vi "StateMachineDAQ-modified.vi"() -> ()   [LabVIEW 2015]
doc: "Use this template to build a user interface event handler design pattern. Use this pattern for dialog boxes and other user interfaces. You also can create and execute user-defined events that the VI can handle the same way as user interface events."
uses:
  StateMachineDAQState.ctl
  <vilib>/Utility/error.llb/DialogType.ctl
  <vilib>/DAQmx/read.llb/DAQmx Read (Analog Wfm 1Chan NSamp).vi
  <vilib>/DAQmx/create/channels.llb/DAQmx Create Channel (AI-Voltage-Basic).vi
  <vilib>/DAQmx/configure/timing.llb/DAQmx Timing (Sample Clock).vi
  <vilib>/DAQmx/miscellaneous.llb/DAQmx Fill In Error Info.vi
  <resource>/objmgr/daqmx.rc
panel:
  in  "Process 1":bool
  in  "File Path":path
  in  "Acquire Data":bool
  in  "Log Data":bool
  in  "File Comment":string
  in  "DAQ Parameters":T1={"physical channels"="", "maximum value"=5.0, "minimum value"=-5.0, "rate"=1000.0, "read period"=0.5} {"read period" format="%0.2f"; "rate" format="%0.2f"; "minimum value" format="%0.2f"; "maximum value" format="%0.2f"}
  out "Waveform Chart":waveform(dbl)(graph)
  in  "quit":bool
  # "V"
  # "V"
  # "Hz"
  # "s"
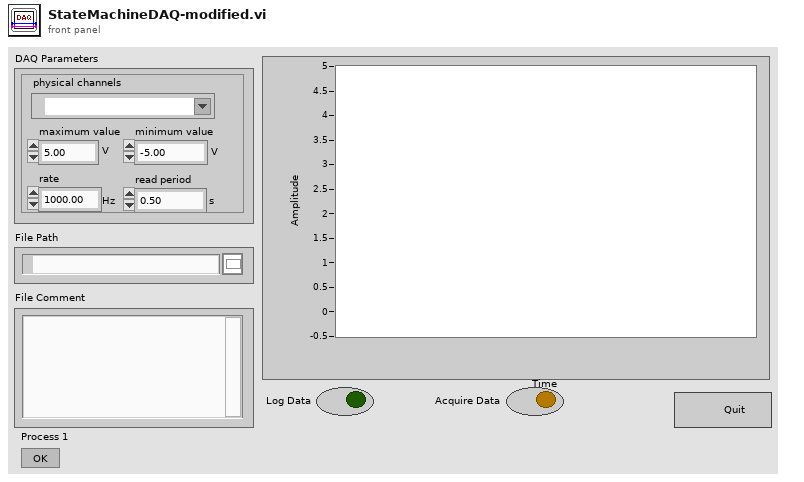
[diagram p1: front panel]
types:
  T1 = cluster{"physical channels":tag, "maximum value":dbl, "minimum value":dbl, "rate":dbl, "read period":dbl}
  T2 = typedef "StateMachineDAQState.ctl" = enum16{"Init", "Idle", "CheckError", "Finalize", "ConfigDAQ", "StartDAQ", "AcquireAndLog", "StopDAQ", "ClearDAQ", "OpenFile", "CloseFile", "Process 1"}
  T3 = typedef "DialogType.ctl" = u16
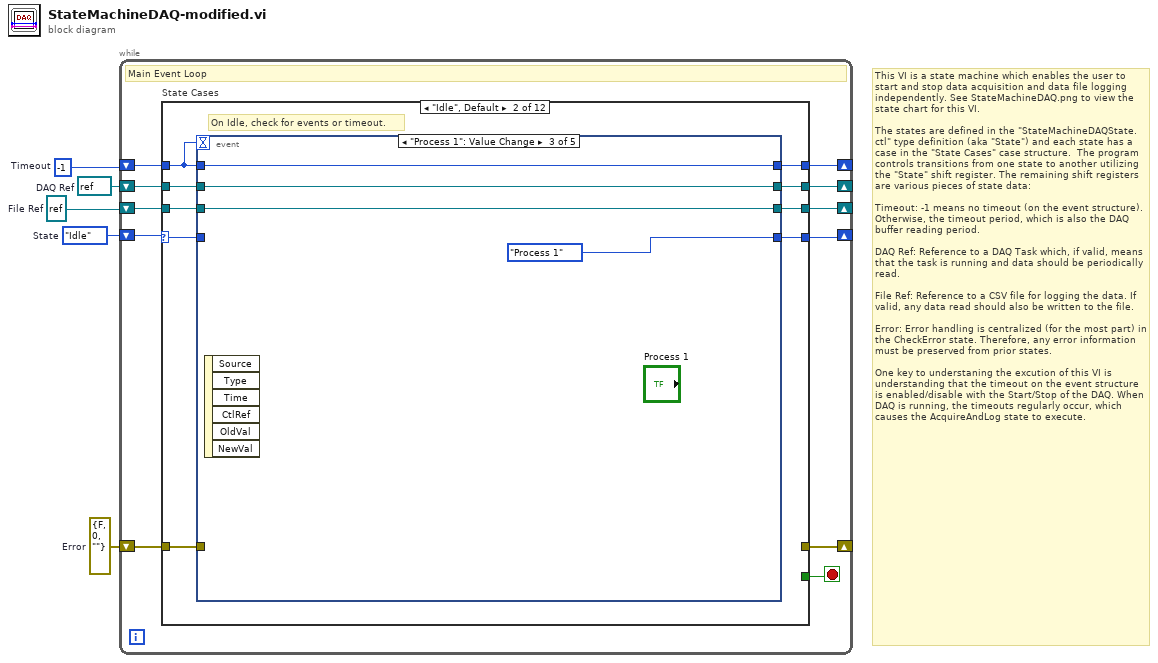
[diagram p0: block diagram]
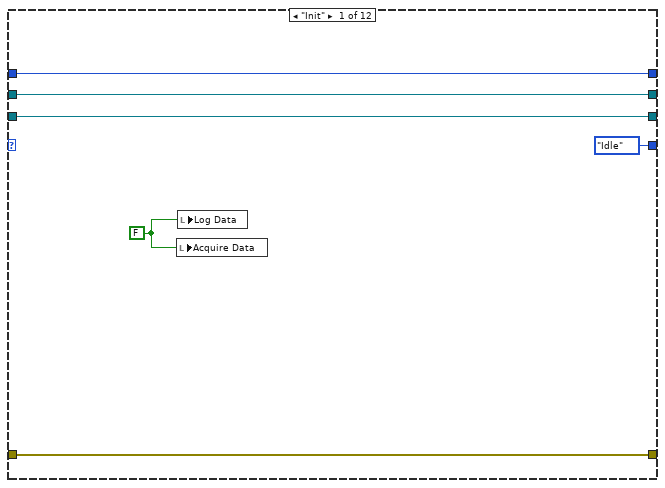
[diagram p2: hidden frame]
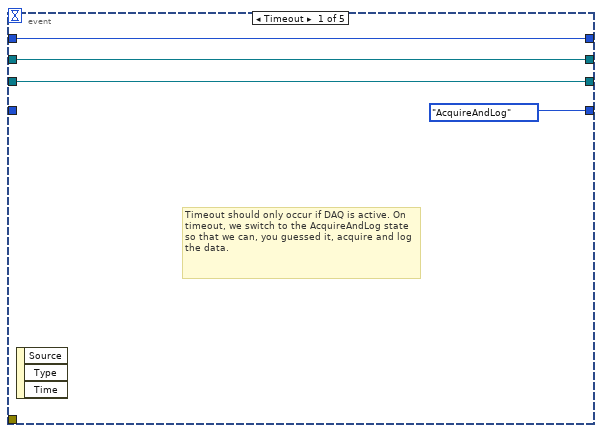
[diagram p3: hidden frame]
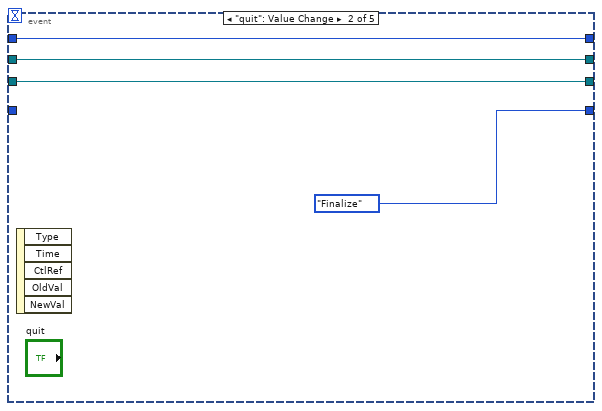
[diagram p4: hidden frame]
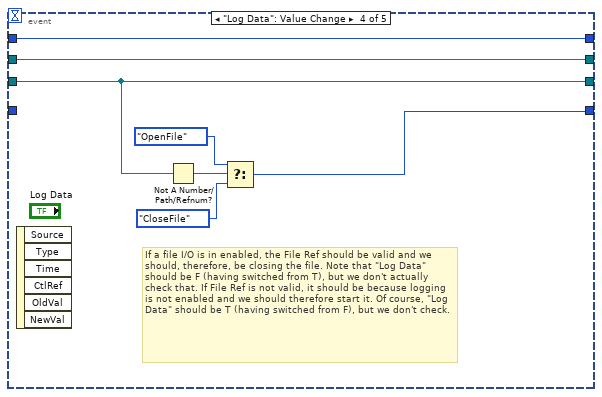
[diagram p5: hidden frame]
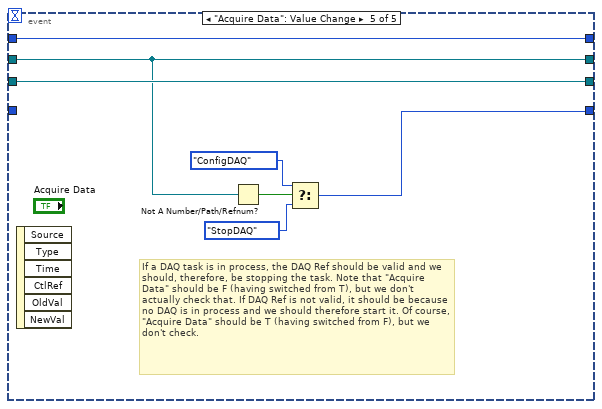
[diagram p6: hidden frame]
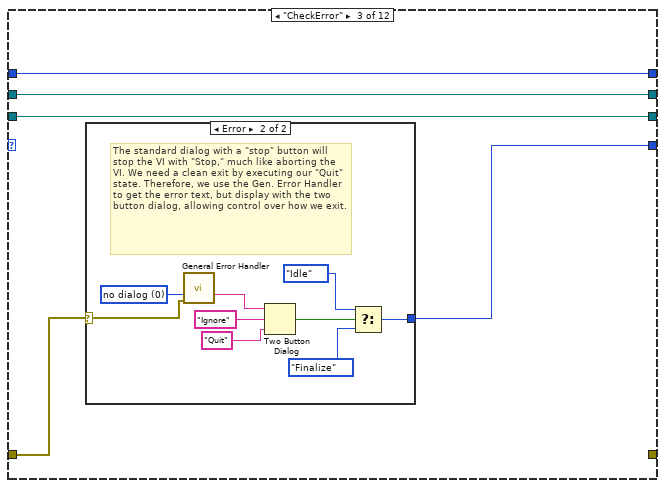
[diagram p7: hidden frame]
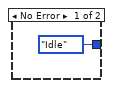
[diagram p8: hidden frame]
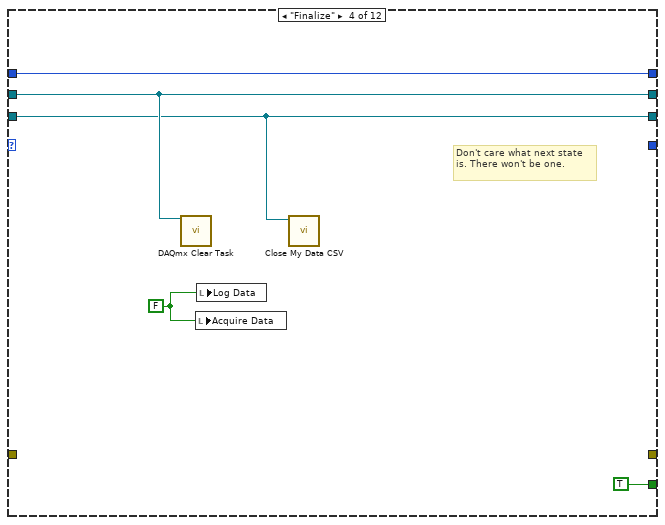
[diagram p9: hidden frame]
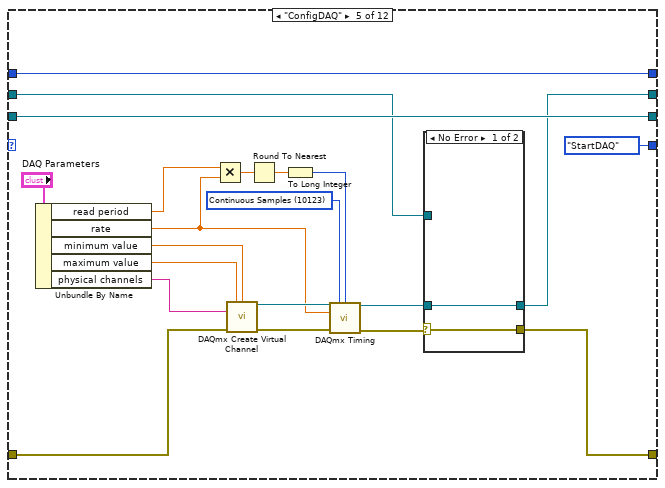
[diagram p10: hidden frame]
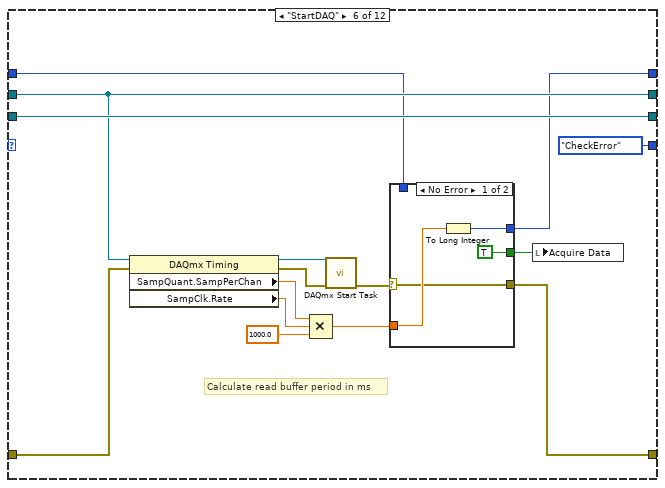
[diagram p12: hidden frame]
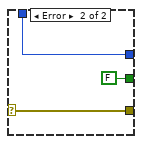
[diagram p13: hidden frame]
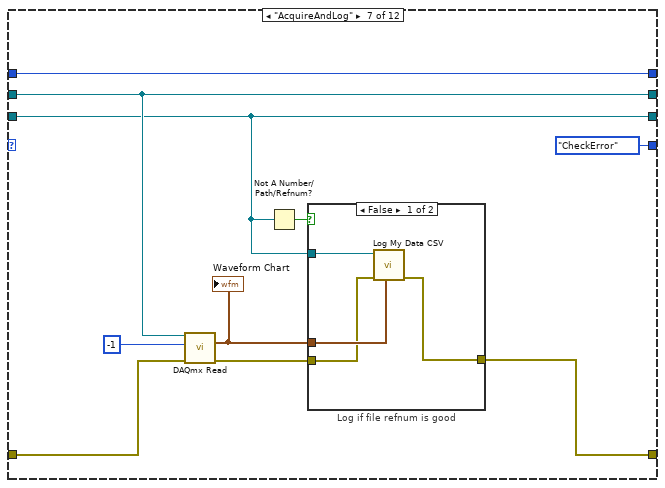
[diagram p14: hidden frame]
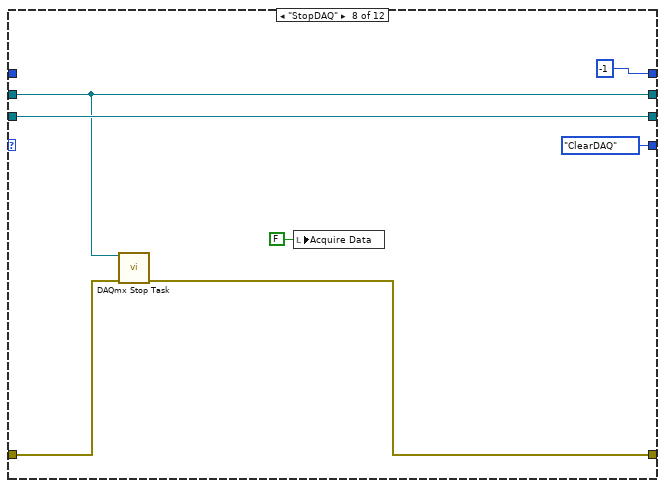
[diagram p16: hidden frame]
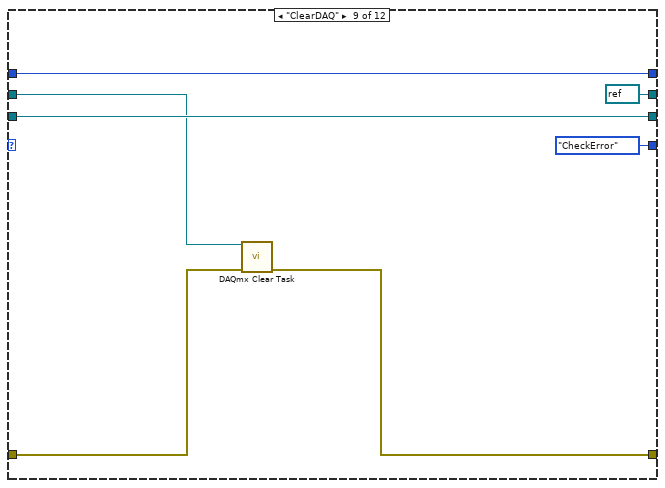
[diagram p17: hidden frame]
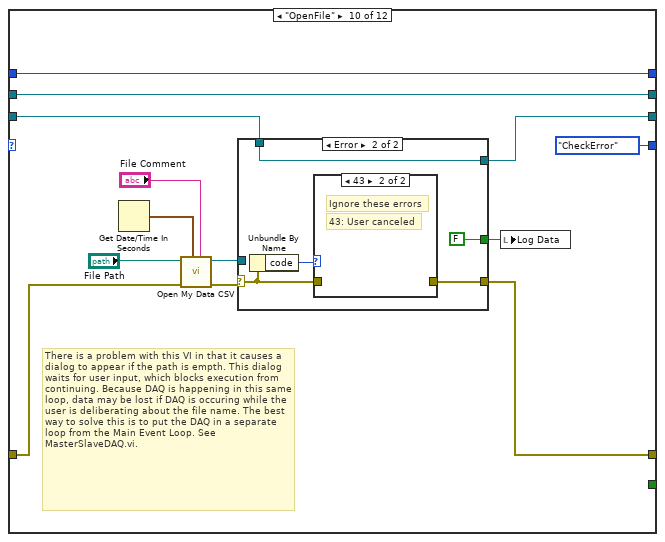
[diagram p18: hidden frame]
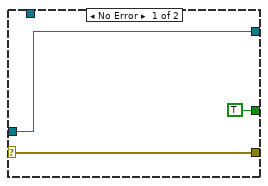
[diagram p19: hidden frame]
diagram:
  w1 = errorcluster {"status"=FALSE, "code"=0, "source"=""}  # Error
  w2 = refnum<file> refnum  # File Ref
  w3 = refnum<k21> refnum  # DAQ Ref
  w4 = StateMachineDAQState."Idle"  # State
  w5 = -1  # Timeout
  # "This VI is a state machine which enables the user to start and stop data acquisition and data file logging independently. See StateMachineDAQ.png to view the state chart for this VI.\n\nThe states are defined in the \"StateMachineDAQState.ctl\" type definition (aka \"State\") and each state has a case in the \"State Cases\" case structure.  The program controls transitions from one state to another utilizing the \"State\" shift register. The remaining shift registers are various pieces of state data:\n\nTimeout: -1 means no timeout (on the event structure). Otherwise, the timeout period, which is also the DAQ buffer reading period.\n\nDAQ Ref: Reference to a DAQ Task which, if valid, means that the task is running and data should be periodically read.\n\nFile Ref: Reference to a CSV file for logging the data. If valid, any data read should also be written to the file.\n\nError: Error handling is centralized (for the most part) in the CheckError state. Therefore, any error information must be preserved from prior states.\n\nOne key to understaning the excution of this VI is understanding that the timeout on the event structure is enabled/disable with the Start/Stop of the DAQ. When DAQ is running, the timeouts regularly occur, which causes the AcquireAndLog state to execute."
  n1 = while {
    shift-right: [w15] -> _
    shift-left: w5 -> [w16]
    shift-right: [w13] -> _
    shift-left: w4 -> [w14]
    shift-right: [w12] -> _
    shift-left: w3 -> [w11]
    shift-right: [w10] -> _
    shift-left: w2 -> [w9]
    shift-right: [w8] -> _
    shift-left: w1 -> [w7]
    stop <- w6 stop-if-true
    # "Main Event Loop"
    n2 = case "State Cases" shown="\"Idle\", Default" w14 {
      selector: w14 -> [_ w29 _ _ _ _ _ _ _ _ _ _]
      tunnel: w16 -> [w22 w31 w62 w77 w86 w112 w130 _ w153 w166 w183 w190]
      tunnel: [w22 w30 w62 w77 w86 w111 w130 -1 ("Timeout") w153 w166 w183 w190] -> w15
      tunnel: [StateMachineDAQState."Idle" ("State") w28 w59 _ StateMachineDAQState."StartDAQ" ("State") StateMachineDAQState."CheckError" ("State") StateMachineDAQState."CheckError" ("State") StateMachineDAQState."ClearDAQ" ("State") StateMachineDAQState."CheckError" ("State") StateMachineDAQState."CheckError" ("State") w176 StateMachineDAQState."CheckError" ("State")] -> w13
      tunnel: [w21 w25 w61 w75 w89 w116 w129 w141 refnum<k21> refnum ("DAQ Ref") w165 w182 w189] -> w12
      tunnel: w11 -> [w21 w24 w61 w75 w90 w116 w129 w141 w149 w165 w182 w189]
      tunnel: [w20 w27 w60 w74 w98 w117 w128 w146 w151 w159 w179 w188] -> w10
      tunnel: w9 -> [w20 w26 w60 w74 w98 w117 w128 w146 w151 w154 w181 _]
      tunnel: [w17 _ _ _ w87 w110 w127 w142 w147 w158 _ _] -> w8
      tunnel: w7 -> [w17 w23 w58 _ w78 w107 w125 w140 w148 w155 w178 _]
      tunnel: [_ _ _ TRUE _ _ _ _ _ _ _ _] -> w6
      frame "Init" {
        w18 = FALSE
        n3 = local write "Acquire Data"(w18) -> ()
        n4 = local write "Log Data"(w18) -> ()
      }
      frame "Idle", Default {
        # "On Idle, check for events or timeout."
        # "States"
        n5 = event shown="[2] \"Process 1\": Value Change" {
          selector: _ -> [_ _ _ _ _]
          dyn-events: _ -> [_ _ _ _ _]
          timeout: w31 -> [_ _ _ _ _]
          tunnel: w31 -> [w35 w39 w42 w50 w57]
          tunnel: [w35 w39 w42 w50 w57] -> w30
          tunnel: w29 -> [_ _ _ _ _]
          tunnel: [StateMachineDAQState."AcquireAndLog" ("State") StateMachineDAQState."Finalize" ("State") StateMachineDAQState."Process 1" ("State") w44 w51] -> w28
          tunnel: [w32 w37 w40 w47 w56] -> w27
          tunnel: w26 -> [w32 w37 w40 w47 w56]
          tunnel: [w34 w38 w41 w49 w54] -> w25
          tunnel: w24 -> [w34 w38 w41 w49 w54]
          tunnel: w23 -> [_ _ _ _ _]
          event Timeout {
            # "Timeout should only occur if DAQ is active. On timeout, we switch to the AcquireAndLog state so that we can, you guessed it, acquire and log the data."
            n6 = event-data() -> ()  [unwired: 1 in, 3 out]
          }
          event "quit": Value Change {
            n7 = event-data() -> ()  [unwired: 1 in, 5 out]
          }
          event "Process 1": Value Change {
            n8 = event-data() -> ()  [unwired: 1 in, 6 out]
          }
          event "Log Data": Value Change {
            # "If a file I/O is in enabled, the File Ref should be valid and we should, therefore, be closing the file. Note that \"Log Data\" should be F (having switched from T), but we don't actually check that. If File Ref is not valid, it should be because logging is not enabled and we should therefore start it. Of course, \"Log Data\" should be T (having switched from F), but we don't check."
            n9 = event-data() -> ()  [unwired: 1 in, 6 out]
            n10 = Not A Number/Path/Refnum?(number/path/refnum=w47) -> (NaN/Path/Refnum?=w48:bool)
            n11 = Select(t=StateMachineDAQState."OpenFile" ("State"), s=w48, f=StateMachineDAQState."CloseFile" ("State")) -> (s? t:f=w44:T2)
          }
          event "Acquire Data": Value Change {
            # "If a DAQ task is in process, the DAQ Ref should be valid and we should, therefore, be stopping the task. Note that \"Acquire Data\" should be F (having switched from T), but we don't actually check that. If DAQ Ref is not valid, it should be because no DAQ is in process and we should therefore start it. Of course, \"Acquire Data\" should be T (having switched from F), but we don't check."
            n12 = event-data() -> ()  [unwired: 1 in, 6 out]
            n13 = Not A Number/Path/Refnum?(number/path/refnum=w54) -> (NaN/Path/Refnum?=w55:bool)
            n14 = Select(t=StateMachineDAQState."ConfigDAQ" ("State"), s=w55, f=StateMachineDAQState."StopDAQ" ("State")) -> (s? t:f=w51:T2)
          }
        }
      }
      frame "CheckError" {
        n15 = case shown="Error" w58 {
          selector: w58 -> [_ w64]
          tunnel: [StateMachineDAQState."Idle" ("State") w65] -> w59
          frame No Error {
          }
          frame Error {
            w72 = T3 0 items=["no dialog", "OK message", "continue or stop message", "OK message + warnings", "continue/stop + warnings"] ("type of dialog (OK msg:1)")
            # "The standard dialog with a \"stop\" button will stop the VI with \"Stop,\" much like aborting the VI. We need a clean exit by executing our \"Quit\" state. Therefore, we use the Gen. Error Handler to get the error text, but display with the two button dialog, allowing control over how we exit."
            n16 = call <vilib>:"General Error Handler.vi"("type of dialog (OK msg:1)"=w72, "error in (no error)"=w64) -> ("message"=w71:string)  [unwired: 9 in, 4 out]
            n17 = Two Button Dialog(message=w71, 1:"Quit" ("F button name (\"Cancel\")"), 2:"Ignore" ("T button name (\"OK\")")) -> (T button?=w68:bool)
            n18 = Select(t=StateMachineDAQState."Idle" ("State"), s=w68, f=StateMachineDAQState."Finalize" ("State")) -> (s? t:f=w65:T2)
          }
        }
      }
      frame "Finalize" {
        w73 = FALSE
        # "Don't care what next state is. There won't be one."
        n19 = call <vilib>:"DAQmx Clear Task.vi"("task in"=w75) -> ()  [unwired: 14 in, 1 out]
        n20 = local write "Acquire Data"(w73) -> ()
        n21 = local write "Log Data"(w73) -> ()
        n22 = call "Close My Data CSV.vi"("file refnum"=w74) -> ()  [unwired: 10 in, 1 out]
      }
      frame "ConfigDAQ" {
        w95 = 10123 items=["Finite Samples"=10178, "Continuous Samples"=10123, "Hardware Timed Single Point"=12522] ("sample mode")
        n23 = Unbundle By Name("DAQ Parameters") -> ("read period"=w83:dbl, "rate"=w82:dbl, "minimum value"=w81:dbl, "maximum value"=w80:dbl, "physical channels"=w79:tag)
        n24 = Multiply(x=w83, y=w82) -> (x*y=w94:dbl)
        n25 = call-poly <vilib>:"DAQmx Create Virtual Channel.vi"("maximum value"=w80, "minimum value"=w81, "physical channels"=w79, "error in"=w78) -> ("task out"=w97:refnum<k21>, "error out"=w96:errorcluster)  [unwired: 10 in]
        n26 = Round To Nearest(number=w94) -> (nearest integer value=w93:dbl)
        n27 = To Long Integer(number=w93) -> (32bit integer=w92:i32)
        n28 = call-poly <vilib>:"DAQmx Timing.vi"("task/channels in"=w97, "sample mode"=w95, "samples per channel"=w92, "rate"=w82, "error in"=w96) -> ("task out"=w88:refnum<k21>, "error out"=w91:errorcluster)  [unwired: 9 in]
        n29 = case shown="No Error" w91 {
          selector: w91 -> [w99 w102]
          tunnel: w90 -> [_ w101]
          tunnel: [w100 w101] -> w89
          tunnel: w88 -> [w100 _]
          tunnel: [w99 w102] -> w87
          frame No Error {
          }
          frame Error {
          }
        }
      }
      frame "StartDAQ" {
        # "Calculate read buffer period in ms"
        n30 = property class="DAQmx Timing"(reference=w116, error in=w107) -> (reference out=w115:refnum<k21>, error out=w114:errorcluster, "SampQuant.SampPerChan"=w106:dbl, "SampClk.Rate"=w105:dbl)
        n31 = Compound Arithmetic op=MULTIPLY(w106, w105, 1000.0 ("value")) -> (w103:dbl)
        n32 = call <vilib>:"DAQmx Start Task.vi"("task/channels in"=w115, "error in"=w114) -> ("error out"=w113:errorcluster)  [unwired: 12 in, 1 out]
        n33 = case shown="No Error" w113 {
          selector: w113 -> [w119 w123]
          tunnel: w103 -> [w121 _]
          tunnel: w112 -> [_ w124]
          tunnel: [w120 w124] -> w111
          tunnel: [w119 w123] -> w110
          tunnel: [TRUE FALSE] -> w108
          frame No Error {
            n34 = To Long Integer(number=w121) -> (32bit integer=w120:i32)
          }
          frame Error {
          }
        }
        n35 = local write "Acquire Data"(w108) -> ()
      }
      frame "AcquireAndLog" {
        n36 = call-poly <vilib>:"DAQmx Read.vi"("task/channels in"=w129, "number of samples per channel"=-1, "error in"=w125) -> ("data"=w131:waveform(dbl), "error out"=w132:errorcluster)  [unwired: 10 in, 1 out]
        "Waveform Chart" <- w131
        n37 = Not A Number/Path/Refnum?(number/path/refnum=w128) -> (NaN/Path/Refnum?=w133:bool)
        n38 = case "Log if file refnum is good" shown="False" w133 {
          tunnel: w132 -> [w136 w139]
          tunnel: w128 -> [w138 _]
          tunnel: w131 -> [w137 _]
          tunnel: [w135 w139] -> w127
          frame False {
            n39 = call "Log My Data CSV.vi"("Data"=w137, "error in"=w136, "file refnum"=w138) -> ("error out"=w135:errorcluster)  [unwired: 7 in, 1 out]
          }
          frame True {
          }
        }
      }
      frame "StopDAQ" {
        n40 = call <vilib>:"DAQmx Stop Task.vi"("task/channels in"=w141, "error in"=w140) -> ("error out"=w142:errorcluster)  [unwired: 12 in, 1 out]
        n41 = local write "Acquire Data"(FALSE ("Acquire Data")) -> ()
      }
      frame "ClearDAQ" {
        n42 = call <vilib>:"DAQmx Clear Task.vi"("task in"=w149, "error in"=w148) -> ("error out"=w147:errorcluster)  [unwired: 13 in]
      }
      frame "OpenFile" {
        # "There is a problem with this VI in that it causes a dialog to appear if the path is empth. This dialog waits for user input, which blocks execution from continuing. Because DAQ is happening in this same loop, data may be lost if DAQ is occuring while the user is deliberating about the file name. The best way to solve this is to put the DAQ in a separate loop from the Main Event Loop. See MasterSlaveDAQ.vi."
        n43 = Get Date/Time In Seconds() -> (seconds since 1Jan1904=w164:timestamp)
        n44 = call "Open My Data CSV.vi"("Comment"="File Comment", "Time Stamp"=w164, "error in"=w155, "file path"="File Path") -> ("error out"=w161:errorcluster, "refnum out"=w160:refnum<file>)  [unwired: 6 in]
        n45 = case shown="Error" w161 {
          selector: w161 -> [w168 w171]
          tunnel: [w169 w173] -> w159
          tunnel: w160 -> [w169 _]
          tunnel: [w168 w170] -> w158
          tunnel: [TRUE ("Log Data") FALSE ("Log Data")] -> w157
          tunnel: w154 -> [_ w173]
          frame No Error {
          }
          frame Error {
            n46 = Unbundle By Name(w171) -> ("code"=w172:i32)
            n47 = case shown="43" w172 {
              tunnel: w171 -> [w175 _]
              tunnel: [w175 _] -> w170
              frame 1, Default {
                # "Process these errors"
              }
              frame 43 {
                # "43: User canceled"
                # "Ignore these errors"
              }
            }
          }
        }
        n48 = local write "Log Data"(w157) -> ()
      }
      frame "CloseFile" {
        w179 = refnum<file> refnum  # File Ref
        n49 = call "Close My Data CSV.vi"("error in"=w178, "file refnum"=w181) -> ("error out"=w177:errorcluster)  [unwired: 9 in]
        n50 = local write "Log Data"(FALSE ("Log Data")) -> ()
        n51 = case shown="Error" w177 {
          tunnel: [StateMachineDAQState."Process 1" ("State") StateMachineDAQState."CheckError" ("State")] -> w176
          frame No Error {
          }
          frame Error {
          }
        }
      }
      frame "Process 1" {
        w188 = refnum<file> refnum  # File Ref
        n52 = One Button Dialog(message="Blocking Process") -> ()  [unwired: 1 in, 1 out]
      }
    }
  }
